vi "start.vi"(0 "TestSeries in":refnum<class "TestSeries.lvclass">, 5 "Serial Number":string, 7 "Operator":string, 9 "Comments":string, 11 "error in (no error)":errorcluster) -> (4 "TestSeries out":refnum<class "TestSeries.lvclass">, 15 "error out":errorcluster)   [LabVIEW 2015, in "TestSeries.lvclass"]
uses:
  TestSeries.lvclass
  Typedefs/TestLogTypes.ctl
  Typedefs/TestScenarioTypes.ctl
  TestSeries.lvclass/TestSeries.ctl
  abortTestSeries.vi
  TestLogFactory/ITestLogFactory/ITestLogFactory.lvclass
  TestLog/ITestLog/ITestLog.lvclass
  TestScenarioFactory/ITestScenarioFactory/ITestScenarioFactory.lvclass
  TestScenario/ITestScenario/ITestScenario.lvclass
  Typedefs/ILCBTTypedefs.lvlib
  <userlib>/Common/ILC/ILC/ILC.lvclass
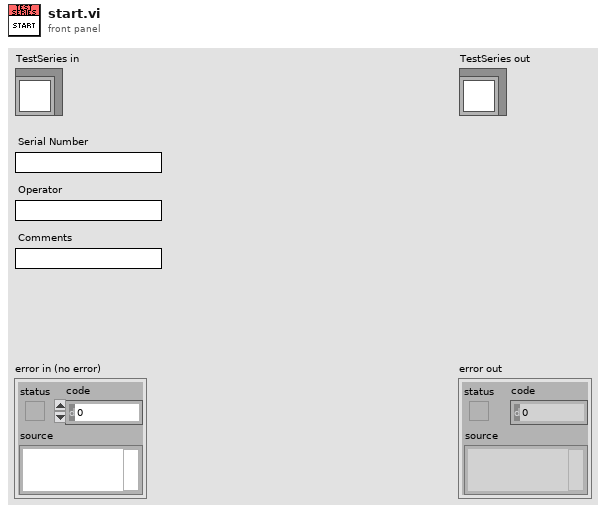
[diagram p1: front panel]
types:
  T1 = typedef "ILCBTTypedefs.lvlib/TestLogTypes.ctl" = enum16{"CSV Test Log"}
  T2 = typedef "ILCBTTypedefs.lvlib/TestScenarioTypes.ctl" = enum16{"+3.3VA Supply Test", "+3.3VD Supply Test", "+5VA Supply Test", "+5VD Supply Test", "Unique ID Test", "TEDS Status Test", "LIMSW1_TTL Low Test", "LIMSW1_TTL High Test", "LIMSW2_TTL Low Test", "LIMSW2_TTL High Test", "Tachometer Low Test", "Tachometer High Test", "SSR_TTL Low Test", "SSR_TTL High Test", "SM_GPI Low Test", "SM_GPI High Test", "CW Motion Without Limit Test", "CW Motion With Limit Test", "CW Motion With Both Limits Test", "CW Motion on CCW Limit Test", "CCW Motion Without Limit Test", "CCW Motion With Limit Test", "CCW Motion With Both Limits Test", "CCW Motion on CW Limit Test", "RS232-TXD Low Test", "RS232-TXD High Test", "RS232-RTS Low Test", "RS232-RTS High Test", "RS232-RXD Low Test", "RS232-RXD High Test", "RS232-CTS Low Test", "RS232-CTS High Test", "Out_SS Low Test", "Out_SS High Test", "Out_SDI Low Test", "Out_SDI High Test", "Out_SCLK Low Test", "Out_SCLK High Test", "Reset Low Test", "Reset High Test", "1 Channel ADC Test", "3 Channel ADC Test", "5 Channel ADC Test", "Vref Test", "ROT Test", "DAC1 Test", "DAC2 Test", "DAC3 Test", "DAC4 Test", "BIAS Test", "EXC1 Test", "EXC2 Test", "EXC3 Test", "EXC4 Test"}
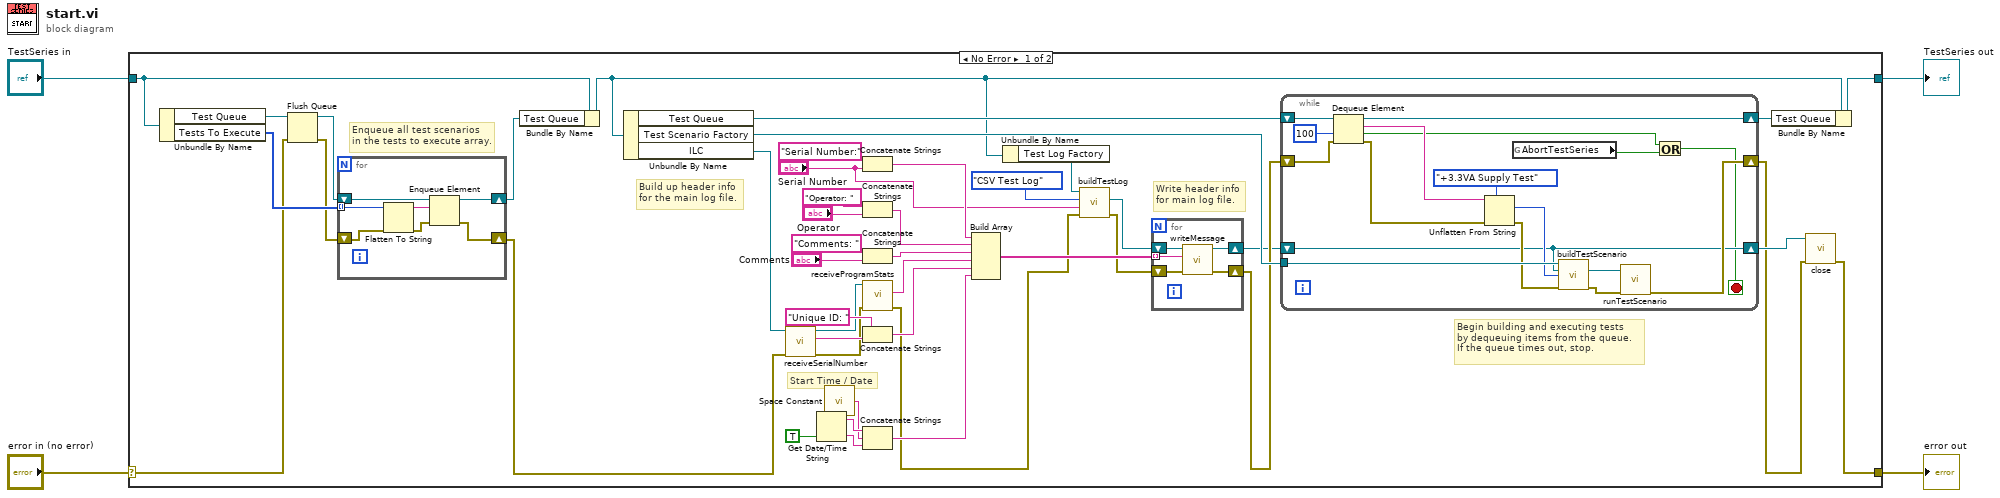
[diagram p0: block diagram]
diagram:
  n1 = case shown="No Error" "error in (no error)" {
    selector: "error in (no error)" -> [w44 w80]
    tunnel: [w6 w80] -> w3
    tunnel: [w40 w79] -> w1
    tunnel: "TestSeries in" -> [w48 w79]
    frame No Error {
      # "Begin building and executing tests\nby dequeuing items from the queue.\nIf the queue times out, stop."
      # "Write header info\nfor main log file."
      # "Build up header info\nfor the main log file."
      # "Enqueue all test scenarios\nin the tests to execute array."
      # "Start Time / Date"
      n2 = Unbundle By Name(w48) -> ("Test Queue"=w49:refnum<queue>, "Tests To Execute"=w47:T2[])
      n3 = Flush Queue(queue=w49, error in (no error)=w44) -> (queue out=w46:refnum<queue>, error out=w43:errorcluster)  [unwired: 1 out]
      n4 = for {
        tunnel: w47 -> [w56] mode=indexing
        shift-right: [w52] -> w45
        shift-left: w46 -> [w54]
        shift-right: [w50] -> w20
        shift-left: w43 -> [w51]
        n5 = Flatten To String(anything=w56, error in (no error)=w51) -> (data string=w55:string, error out=w53:errorcluster)  [unwired: 2 in, 1 out]
        n6 = Enqueue Element(queue=w54, element=w55, error in (no error)=w53) -> (queue out=w52:refnum<queue>, error out=w50:errorcluster)  [unwired: 1 in, 1 out]
      }
      n7 = Bundle By Name(cluster=w48, "Test Queue"=w45) -> (w17:refnum<class "TestSeries.lvclass">)
      n8 = Unbundle By Name(w17) -> ("Test Queue"=w42:refnum<queue>, "Test Scenario Factory"=w18:refnum<class "ITestScenarioFactory.lvclass">, "ILC"=w19:refnum<class "ILC.lvclass">)
      n9 = call <userlib>:"receiveSerialNumber.vi"("error in (no error)"=w20, "ILC in"=w19) -> ("error out"=w31:errorcluster, "Serial Number"=w39:string, "ILC out"=w32:refnum<class "ILC.lvclass">)  [unwired: 7 in]
      n10 = Get Date/Time String(want seconds? (F)=TRUE) -> (date string=w25:string, time string=w5:string)  [unwired: 2 in]
      n11 = call <vilib>:"Space Constant.vi"() -> ("String"=w24:string)
      n12 = Concatenate Strings("Serial Number:" ("string"), "Serial Number") -> (w30:string)
      n13 = Concatenate Strings("Operator: " ("string"), "Operator") -> (w29:string)
      n14 = Concatenate Strings("Comments: " ("string"), "Comments") -> (w28:string)
      n15 = call <userlib>:"receiveProgramStats.vi"("error in (no error)"=w31, "ILC in"=w32) -> ("error out"=w11:errorcluster, "Response"=w27:string)  [unwired: 7 in, 1 out]
      n16 = Concatenate Strings("Unique ID: " ("string"), w39) -> (w26:string)
      n17 = Concatenate Strings(w25, w24, w5) -> (w22:string)
      n18 = Build Array(w30, w29, w28, w27, w26, w22) -> (w21:string[])
      n19 = Unbundle By Name(w17) -> ("Test Log Factory"=w16:refnum<class "ITestLogFactory.lvclass">)
      n20 = call-dynamic "buildTestLog.vi"("error in (no error)"=w11, "Serial Number"="Serial Number", "TestLogTypes"=TestLogTypes."CSV Test Log", "ITestLogFactory in"=w16) -> ("error out"=w12:errorcluster, "ITestLog.lvclass"=w13:refnum<class "ITestLog.lvclass">)  [unwired: 5 in, 1 out]
      n21 = for {
        shift-right: [w57] -> w9
        shift-left: w13 -> [w60]
        tunnel: w21 -> [w59] mode=indexing
        shift-right: [w58] -> w10
        shift-left: w12 -> [w61]
        n22 = call-dynamic "writeMessage.vi"("error in (no error)"=w61, "Message"=w59, "ITestLog in"=w60) -> ("error out"=w58:errorcluster, "ITestLog out"=w57:refnum<class "ITestLog.lvclass">)  [unwired: 7 in]
      }
      n23 = while {
        shift-right: [w77] -> w41
        shift-left: w42 -> [w78]
        shift-right: [w66] -> w7
        shift-left: w10 -> [w75]
        tunnel: w18 -> [w74]
        shift-right: [w65] -> w8
        shift-left: w9 -> [w65]
        stop <- w62 stop-if-true
        n24 = Dequeue Element(queue=w78, timeout in ms (-1)=100, error in (no error)=w75) -> (queue out=w77:refnum<queue>, element=w72:string, timed out?=w63:bool, error out=w70:errorcluster)
        n25 = Unflatten From String(type=TestScenarioTypes."+3.3VA Supply Test" ("Scenario"), binary string=w72, error in (no error)=w70) -> (value=w71:T2, error out=w69:errorcluster)  [unwired: 2 in, 1 out]
        n26 = global read "abortTestSeries.vi" "AbortTestSeries"() -> (w64:bool)
        n27 = call-dynamic "buildTestScenario.vi"("ITestScenarioFactory in"=w74, "Log"=w65, "Test Scenario"=w71, "error in (no error)"=w69) -> ("ITestScenario.lvclass"=w67:refnum<class "ITestScenario.lvclass">, "error out"=w68:errorcluster)  [unwired: 9 in, 1 out]
        n28 = call-dynamic "runTestScenario.vi"("error in (no error)"=w68, "ITestScenario in"=w67) -> ("error out"=w66:errorcluster)  [unwired: 6 in, 3 out]
        n29 = Or(x=w63, y=w64) -> (x .or. y?=w62:bool)
      }
      n30 = Bundle By Name(cluster=w17, "Test Queue"=w41) -> (w40:refnum<class "TestSeries.lvclass">)
      n31 = call-dynamic "close.vi"("error in (no error)"=w7, "ITestLog in"=w8) -> ("error out"=w6:errorcluster)  [unwired: 8 in, 1 out]
    }
    frame Error {
    }
  }
  "error out" <- w3
  "TestSeries out" <- w1
